vi "chromaSendCommend.vi"(4 "Int_Port Timeout":u32=300, 5 "Clu_RemoteOffsetKeylockResult":T3={"Enum_keyLock"=enum."key board lock Off,recall key lock Off", "Enum_Remote/Local"=enum."Go to Local", "Enum_Offset_Get/Off"=enum."Off", "Clu_Result?"={"Byte"=[FALSE, FALSE, TRUE, FALSE, FALSE, FALSE, FALSE, FALSE], "Step"=1}}, 6 "Clu_SysSetting":T2={"Contrast(1~15)"=7, "Buzzer Volume"=enum."High", "EN50191"=enum."Off", "DC50V AGC"=enum."On", "PassOn(0~100)"=0, "End Of Step"=enum."Off", "EOT"=enum."End Of Test"}, 7 "Clus_STDparameter":T4={"EnumFunnction"=enum."Step Parameters", "Hex_DA"=1, "Hex_Master"=50} {"Hex_DA" format="%x"; "Hex_Master" format="%x"}, 8 "ErrIn":errorcluster, 9 "Clu_PresetParameter":T5, 10 "Clu_StepParameters":T6={"Enum_mode"=enum."AC", "StepIndex(1~10)"=1, "RampTime(100ms)"=20, "DwallTime(100ms)"=0, "TestTime(100ms)"=50, "Falltime(100ms)"=30, "HighLimit(100nA)"=10000, "LowLimit(100nA)"=1000, "ArcLimit(100nA)"=10000, "InrushLimit(100nA)"=0, "Sorce(v)"=1000}) -> (0 "ErrOut":errorcluster, 1 "ChecksumError":bool, 2 "Enum_ErrorType":T1, 3 "Str_ ReplyStr":string)   [LabVIEW 2016]
doc: "Include all commend syntax\nSend a message and receive.check checksum \n\n<b>Clu_RemoteOffsetKeyLockResult: </b>\nKeylock\nRemote/Local\nOffset Get/Off\nResult?\n\n<b>Clus_STDparameter:</b>\nMain parameter of every commend\n\n<b>Clu_syssetting:</b>\ncmd systemsetting\n\n<b>Clu_stepParameters</b>\ncmd stepparameters. use bundle by name to set every parameter\n\n<b>Clu_PresetParameter</b>\ncmd presetparameter\n\n<b>Boolean_comerr\nReturn comport error of not\n\n<b>Boolean_ChecksumCurrect</b>\nmanupulate if check sum is currect or not"
uses:
  TypeDef/Enum_ErrorType.ctl
  meter global.vi
panel:
  out "Time_SendNReceive":u32
  out "Boolean_ComErr":bool
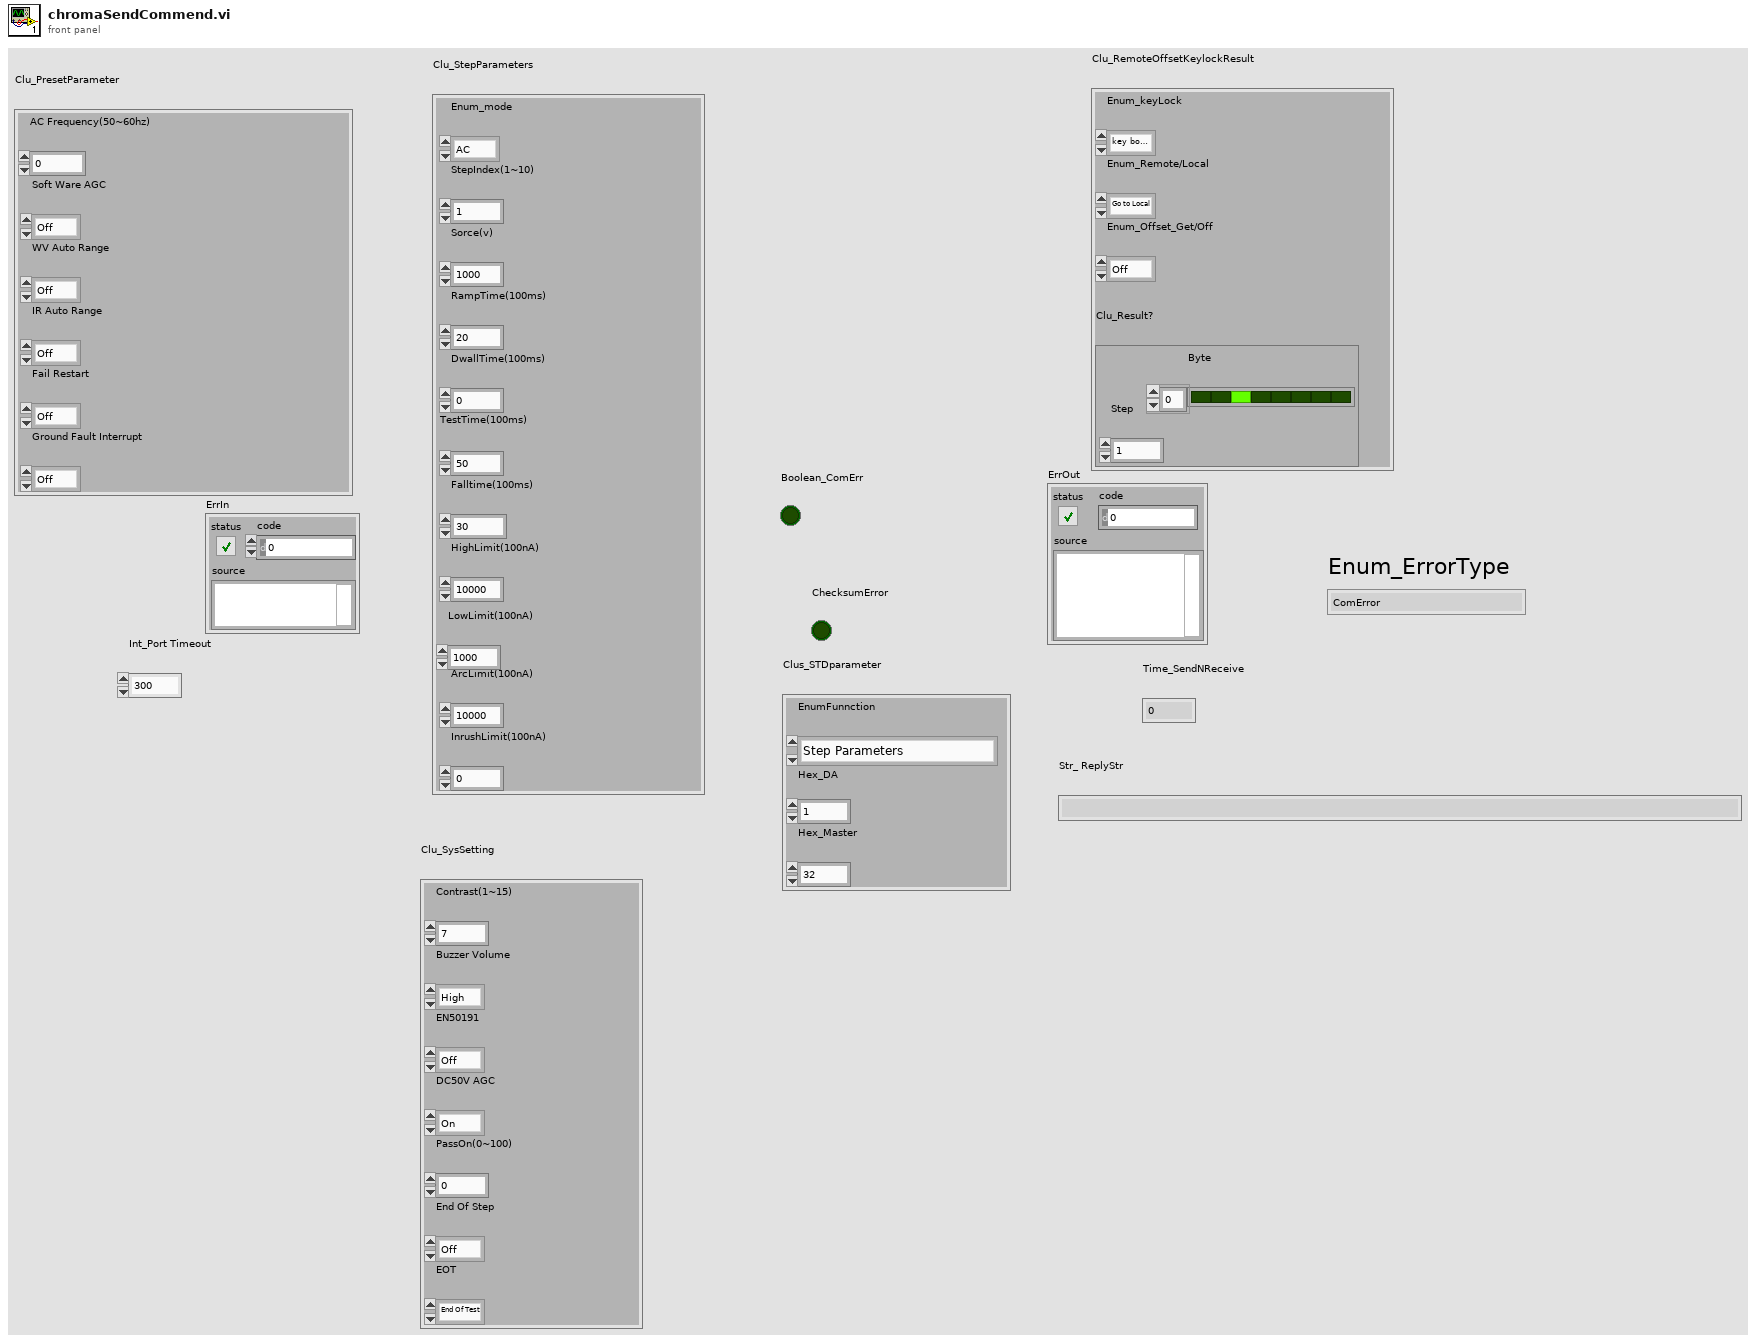
[diagram p1: front panel]
types:
  T1 = typedef "Enum_ErrorType.ctl" = enum16{"ComError", "OK", "Command Error", "Parameter Error"}
  T2 = cluster{"Contrast(1~15)":u8, "Buzzer Volume":enum8{"OFF", "LOW", "Medium", "High"}, "EN50191":enum8{"Off", "On"}, "DC50V AGC":enum8{"Off", "On"}, "PassOn(0~100)":u8, "End Of Step":enum8{"Off", "On"}, "EOT":enum8{"End Of Test", "End Of Timer"}}
  T3 = cluster{"Enum_keyLock":enum8{"key board lock Off,recall key lock Off", "key board lock On,recall key lock Off", "key board lock On,recall key lock On"}, "Enum_Remote/Local":enum8{"Go to Local", "Go to Remote", "Go to Remote and Local Lockout"}, "Enum_Offset_Get/Off":enum8{"Off", "Nonuse", "Get"}, "Clu_Result?":cluster{"Byte":bool[], "Step":u8}}
  T4 = cluster{"EnumFunnction":enum16{"IDN?", "test", "Stop", "Start", "Step Parameters", "Step Patameters?", "Preset Parameter", "Preset parameter?", "Offset Get/Off", "Offset?", "System Setting", "System Setting?", "KeyLock", "KeyLock?", "Initialize All Steps Parameter", "Remote/Local", "Result"}, "Hex_DA":u8, "Hex_Master":u8}
  T5 = cluster{"AC Frequency(50~60hz)":u8, "Soft Ware AGC":enum8{"Off", "On"}, "WV Auto Range":enum8{"Off", "On"}, "IR Auto Range":enum8{"Off", "On"}, "Fail Restart":enum8{"Off", "On"}, "Ground Fault Interrupt":enum8{"Off", "On"}}
  T6 = cluster{"Enum_mode":enum16{"AC", "DC", "IR"}, "StepIndex(1~10)":u8, "RampTime(100ms)":u16, "DwallTime(100ms)":u16, "TestTime(100ms)":u16, "Falltime(100ms)":u16, "HighLimit(100nA)":u32, "LowLimit(100nA)":u32, "ArcLimit(100nA)":u32, "InrushLimit(100nA)":u32, "Sorce(v)":u16}
  T7 = enum8{"Go to Local", "Go to Remote", "Go to Remote and Local Lockout"}
  T8 = enum8{"key board lock Off,recall key lock Off", "key board lock On,recall key lock Off", "key board lock On,recall key lock On"}
  T9 = enum16{"IDN?", "test", "Stop", "Start", "Step Parameters", "Step Patameters?", "Preset Parameter", "Preset parameter?", "Offset Get/Off", "Offset?", "System Setting", "System Setting?", "KeyLock", "KeyLock?", "Initialize All Steps Parameter", "Remote/Local", "Result"}
  T10 = enum16{"big-endian, network order", "native, host order", "little-endian"}
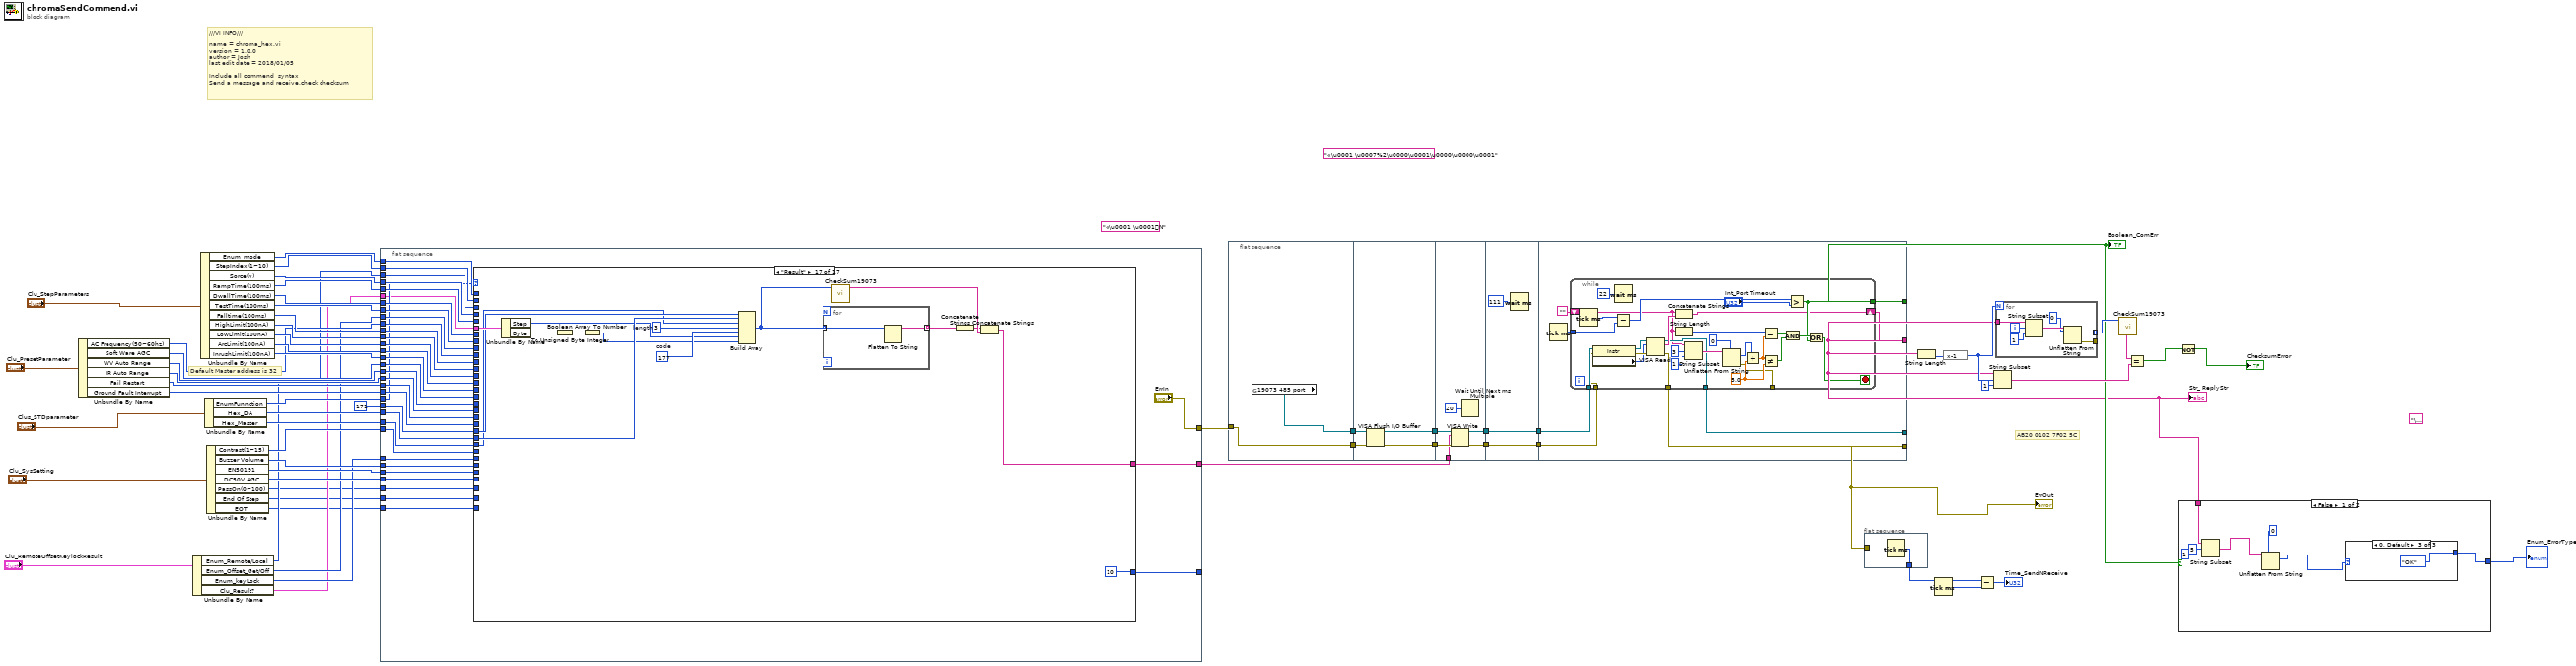
[diagram p0: block diagram]
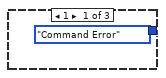
[diagram p2: hidden frame]
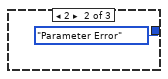
[diagram p3: hidden frame]
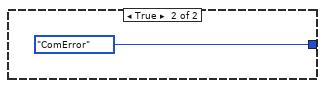
[diagram p4: hidden frame]
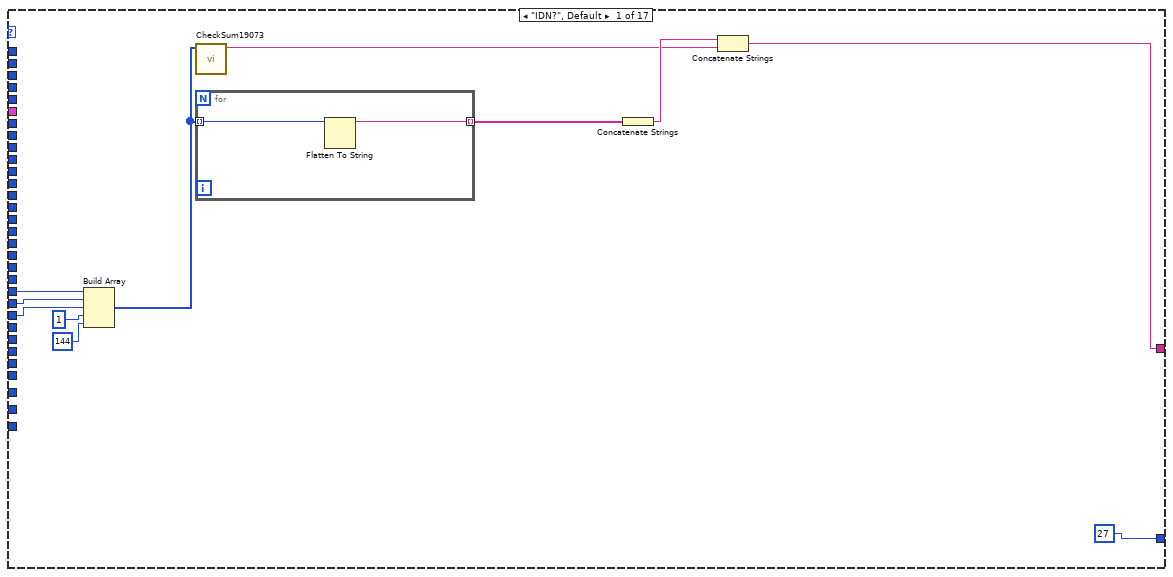
[diagram p5: hidden frame]
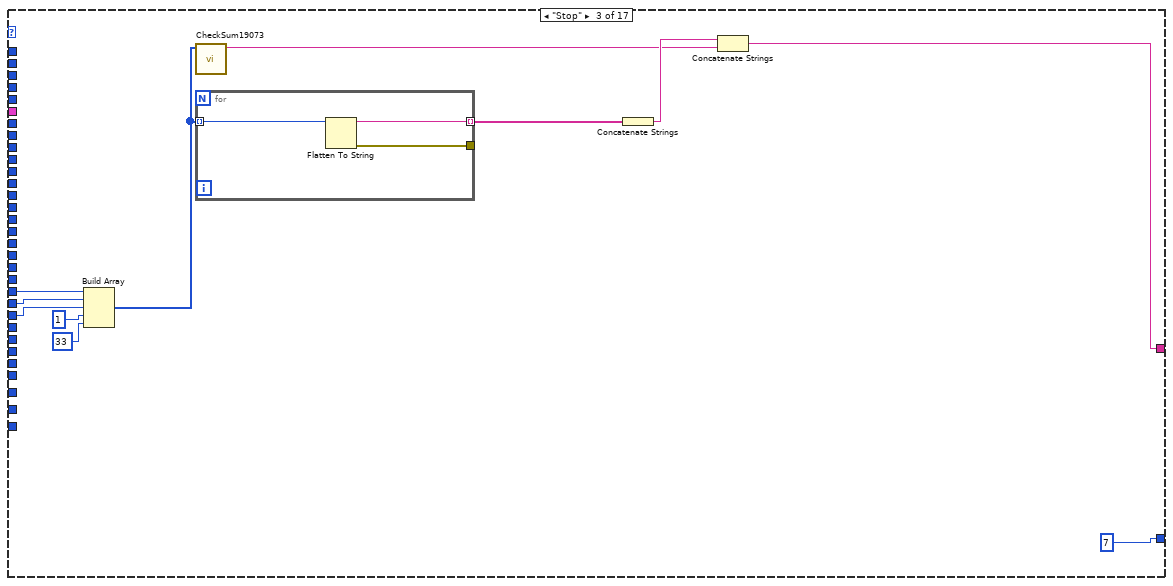
[diagram p7: hidden frame]
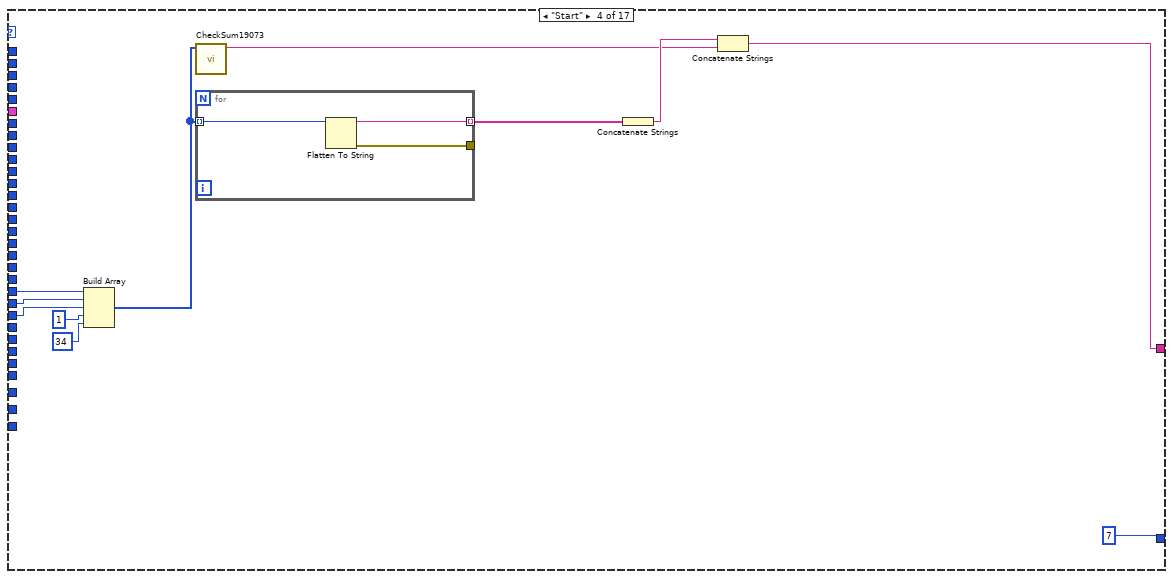
[diagram p8: hidden frame]
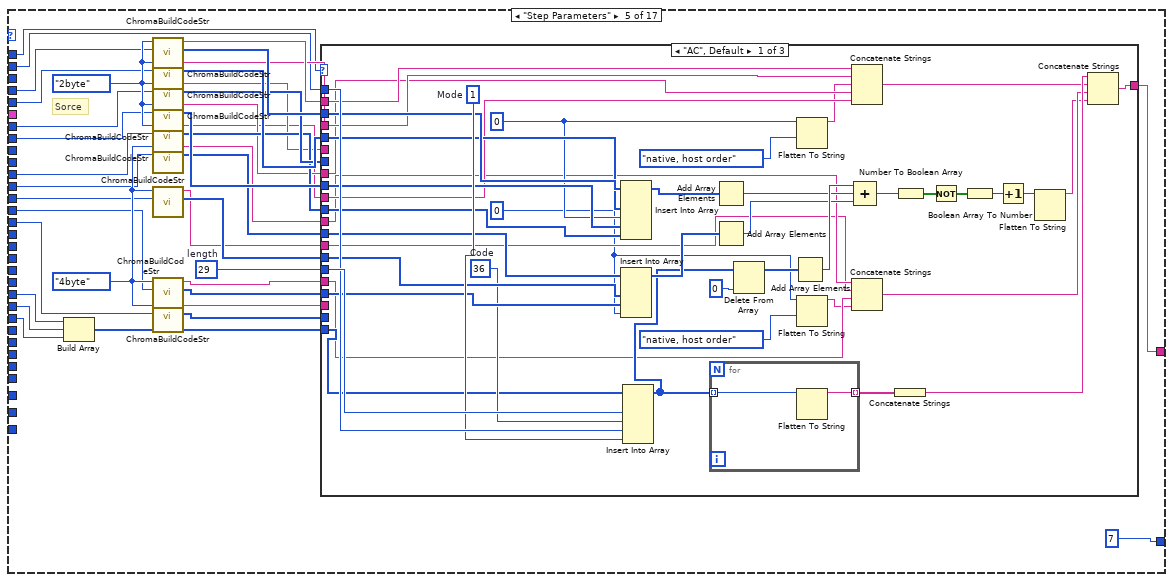
[diagram p9: hidden frame]
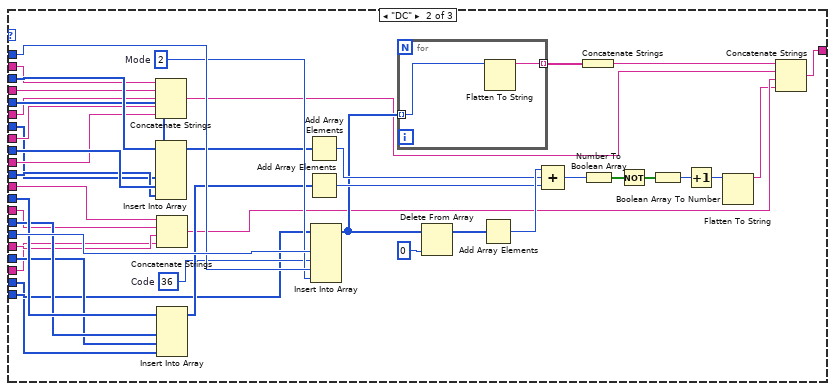
[diagram p10: hidden frame]
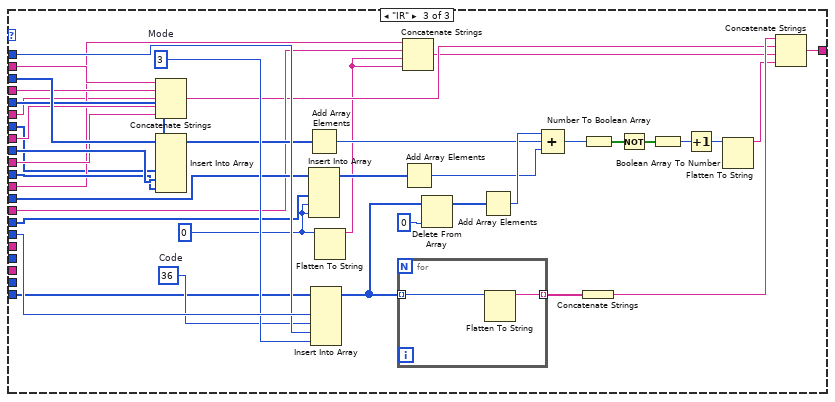
[diagram p11: hidden frame]
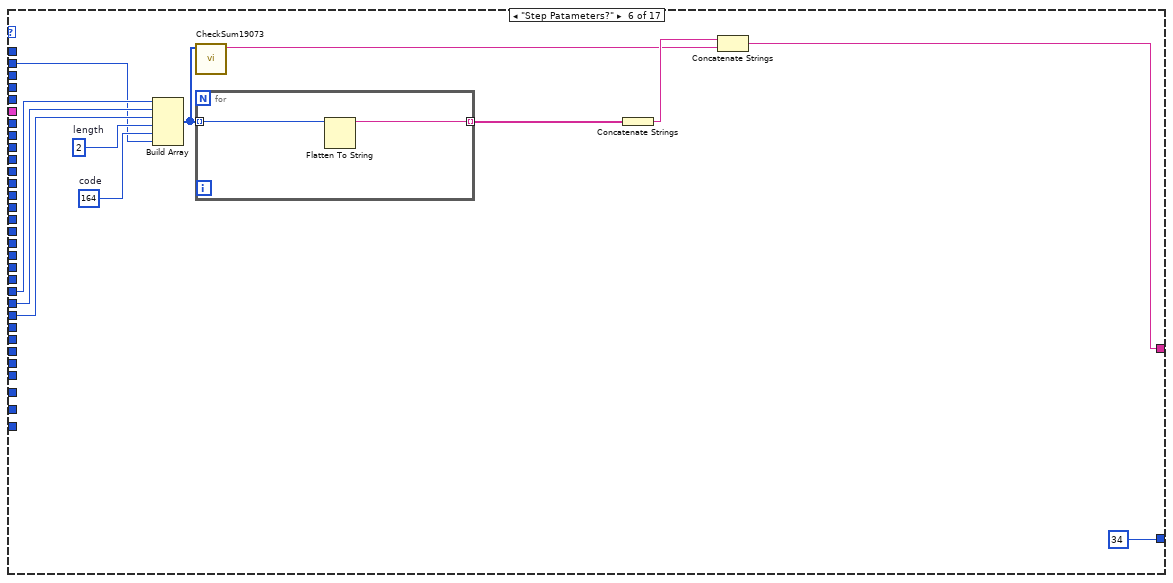
[diagram p12: hidden frame]
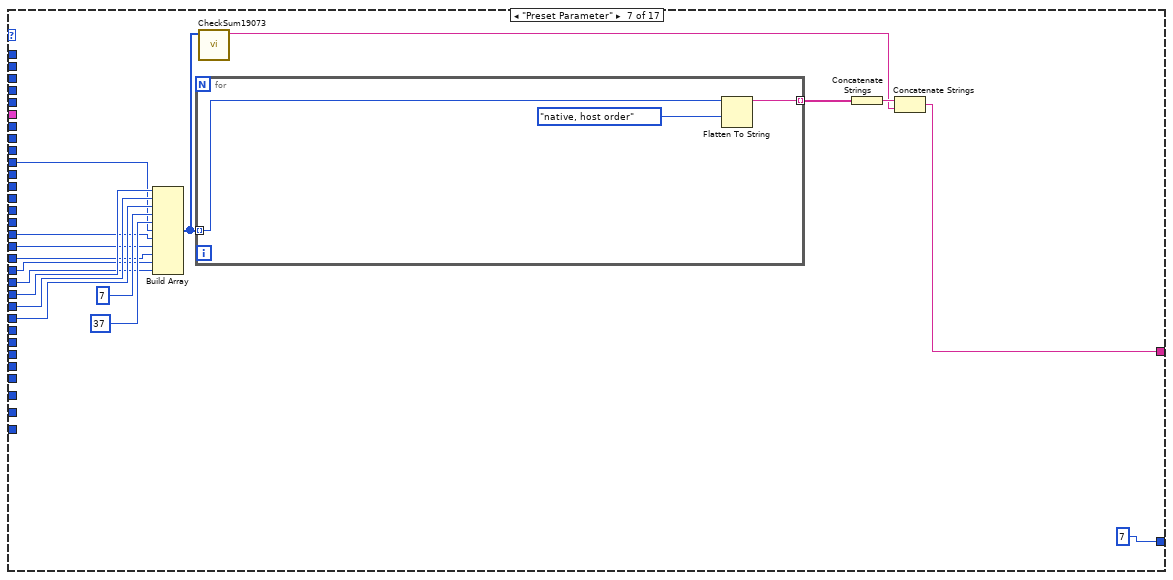
[diagram p13: hidden frame]
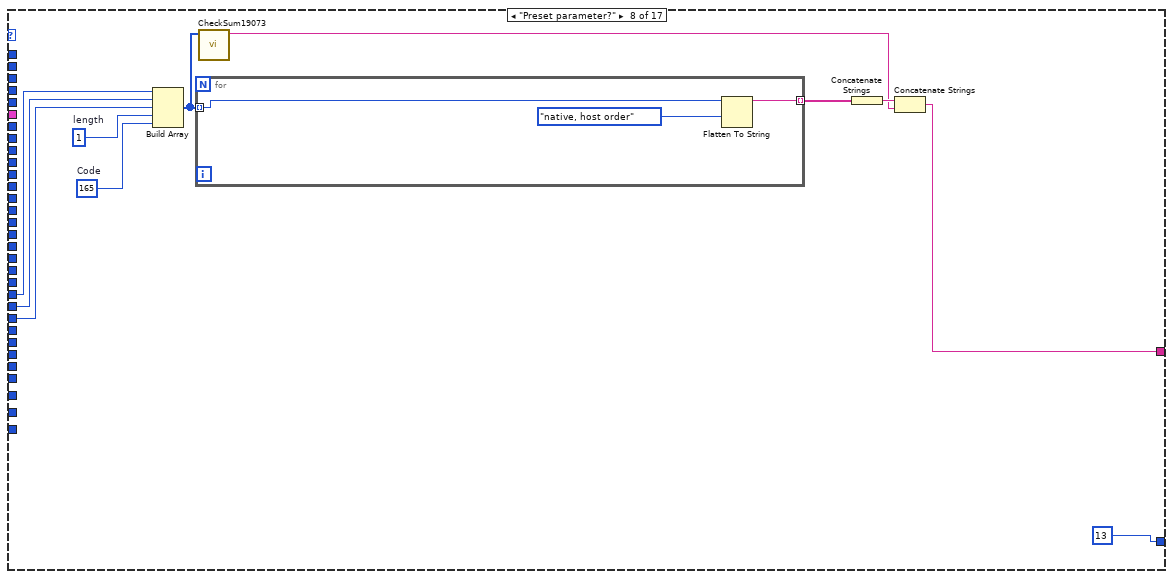
[diagram p14: hidden frame]
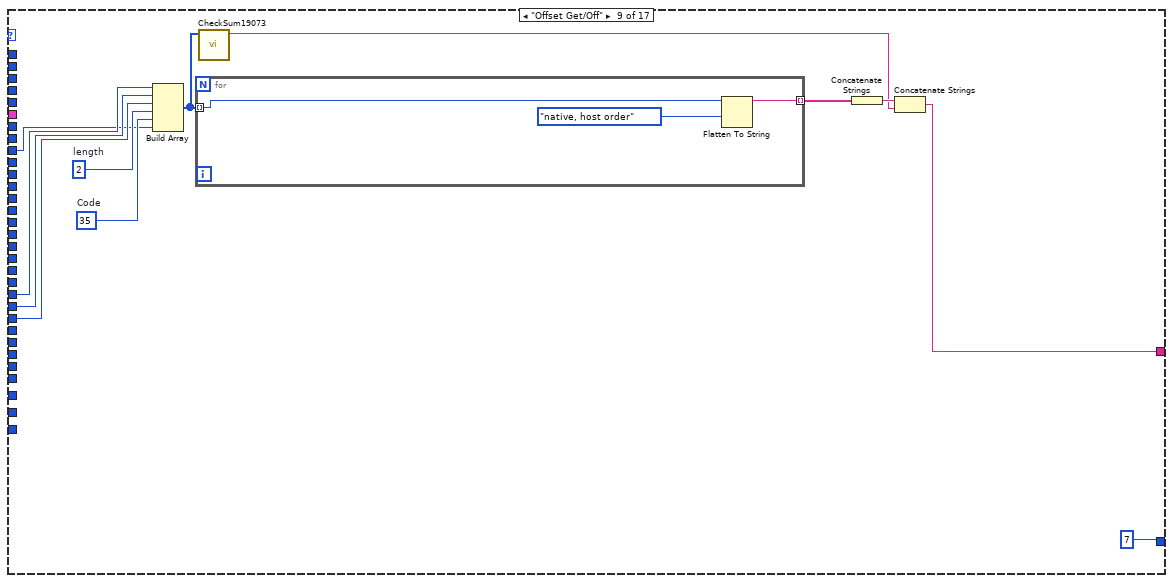
[diagram p15: hidden frame]
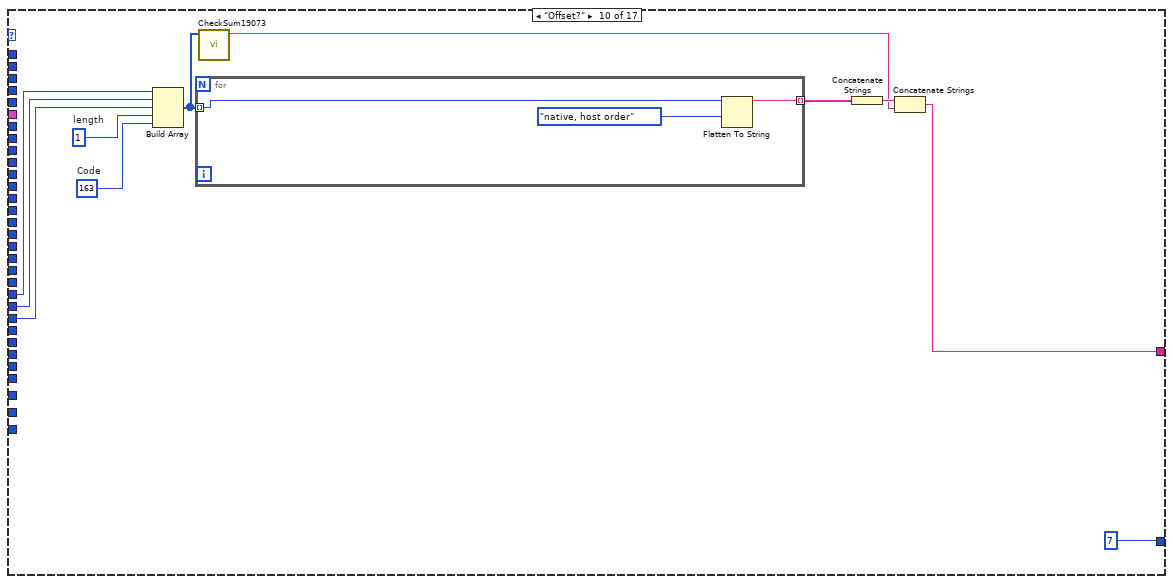
[diagram p16: hidden frame]
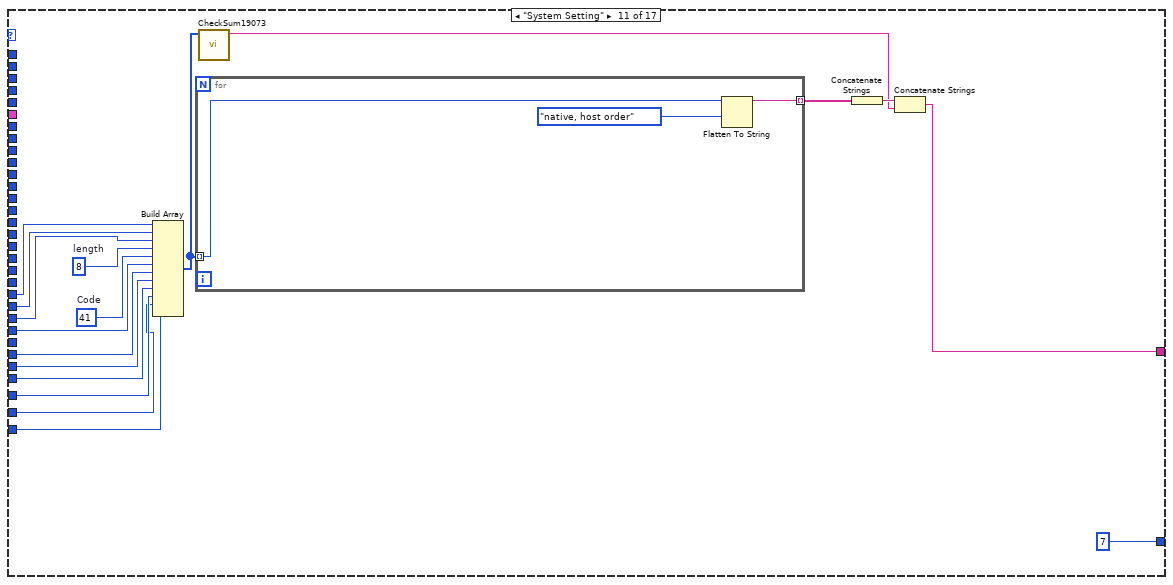
[diagram p17: hidden frame]
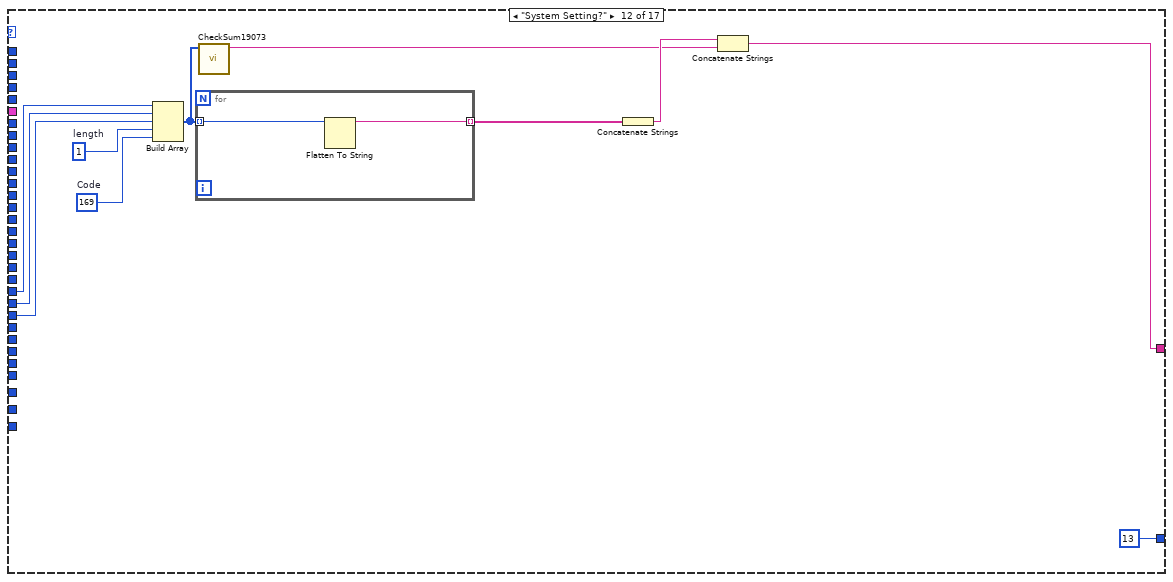
[diagram p18: hidden frame]
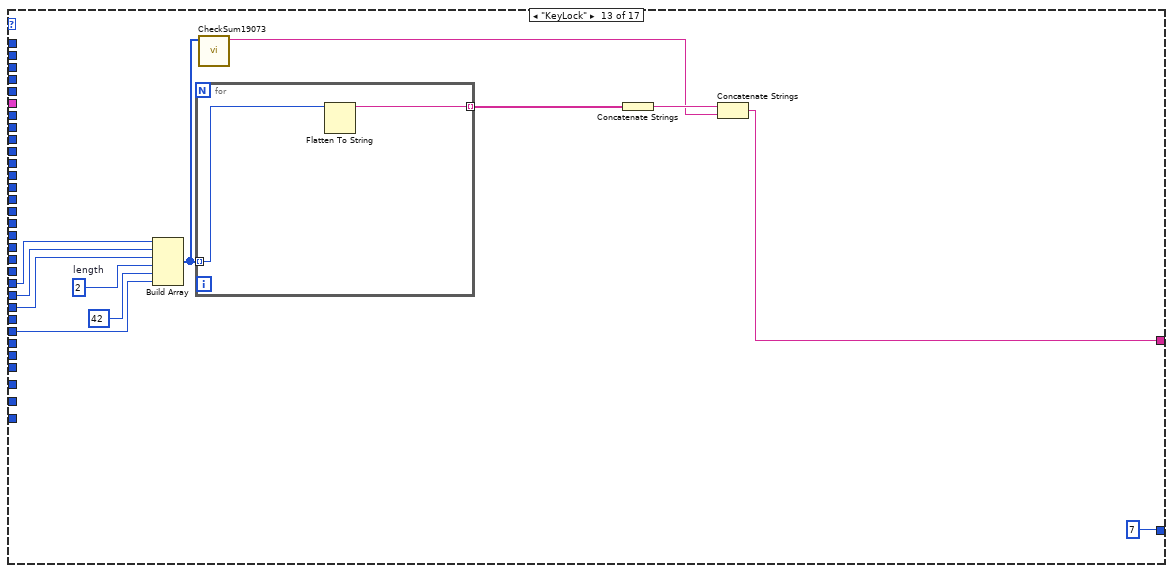
[diagram p19: hidden frame]
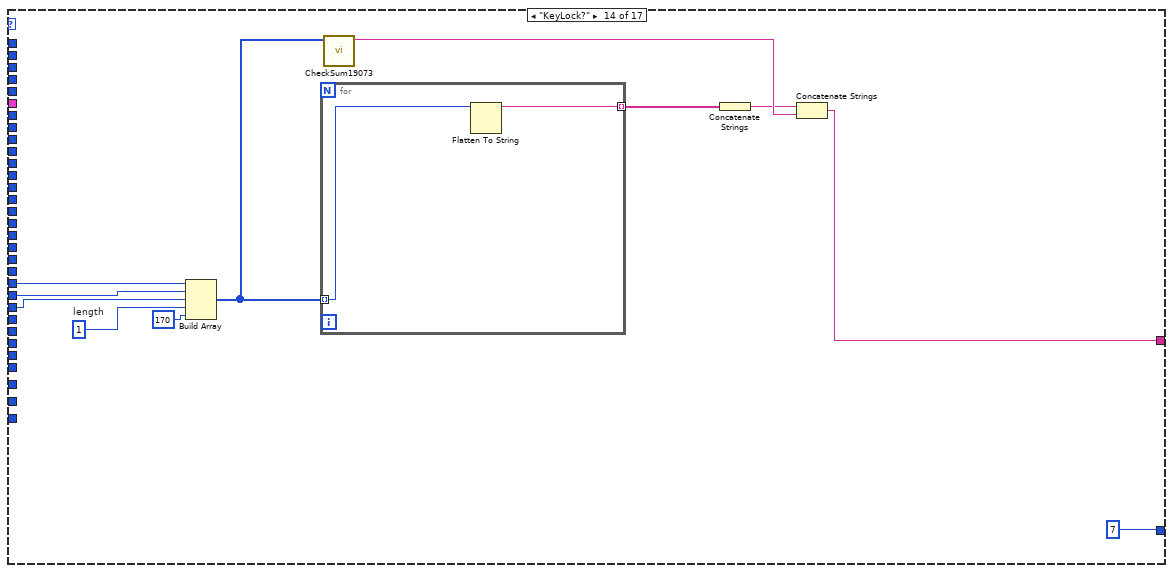
[diagram p20: hidden frame]
diagram:
  (unwired) "\u0002"
  (unwired) "«\u0001 \u0001N" ("Display")
  (unwired) "«\u0001 \u0007%2\u0000\u0001\u0000\u0000\u0001" ("Display")
  # "AB20 0102 7F02 5C"
  # "///VI INFO/// \n\nname = chroma_hex.vi\nversion = 1.0.0\nauthor = Josh\nlast edit date = 2018/01/05\n\nInclude all commend  syntax\nSend a message and receive.check checksum"
  # "Default Master address is 32"
  n1 = Unbundle By Name("Clu_PresetParameter") -> ("AC Frequency(50~60hz)"=w48:u8, "Soft Ware AGC"=w47:enum8{"Off", "On"}, "WV Auto Range"=w46:enum8{"Off", "On"}, "IR Auto Range"=w45:enum8{"Off", "On"}, "Fail Restart"=w44:enum8{"Off", "On"}, "Ground Fault Interrupt"=w43:enum8{"Off", "On"})
  n2 = Unbundle By Name("Clu_RemoteOffsetKeylockResult") -> ("Enum_Remote/Local"=w27:T7, "Enum_Offset_Get/Off"=w26:enum8{"Off", "Nonuse", "Get"}, "Enum_keyLock"=w25:T8, "Clu_Result?"=w21:cluster{"Byte":bool[], "Step":u8})
  n3 = Unbundle By Name("Clu_StepParameters") -> ("Enum_mode"=w60:enum16{"AC", "DC", "IR"}, "StepIndex(1~10)"=w59:u8, "Sorce(v)"=w58:u16, "RampTime(100ms)"=w57:u16, "DwallTime(100ms)"=w56:u16, "TestTime(100ms)"=w55:u16, "Falltime(100ms)"=w54:u16, "HighLimit(100nA)"=w53:u32, "LowLimit(100nA)"=w52:u32, "ArcLimit(100nA)"=w51:u32, "InrushLimit(100nA)"=w50:u32)
  n4 = Unbundle By Name("Clus_STDparameter") -> ("EnumFunnction"=w37:T9, "Hex_DA"=w36:u8, "Hex_Master"=w35:u8)
  n5 = Unbundle By Name("Clu_SysSetting") -> ("Contrast(1~15)"=w42:u8, "Buzzer Volume"=w41:enum8{"OFF", "LOW", "Medium", "High"}, "EN50191"=w40:enum8{"Off", "On"}, "DC50V AGC"=w39:enum8{"Off", "On"}, "PassOn(0~100)"=w19:u8, "End Of Step"=w18:enum8{"Off", "On"}, "EOT"=w17:enum8{"End Of Test", "End Of Timer"})
  n6 = flat-sequence {
    tunnel: u8 171 -> [w97]
    tunnel: w60 -> [w96]
    tunnel: w59 -> [w95]
    tunnel: w58 -> [w94]
    tunnel: w57 -> [w93]
    tunnel: w56 -> [w92]
    tunnel: w55 -> [w91]
    tunnel: w54 -> [w90]
    tunnel: w53 -> [w89]
    tunnel: w52 -> [w88]
    tunnel: w51 -> [w87]
    tunnel: w50 -> [w86]
    tunnel: w48 -> [w85]
    tunnel: w47 -> [w84]
    tunnel: w46 -> [w83]
    tunnel: w45 -> [w82]
    tunnel: w44 -> [w81]
    tunnel: w43 -> [w80]
    tunnel: w26 -> [w79]
    tunnel: w42 -> [w78]
    tunnel: w41 -> [w77]
    tunnel: w40 -> [w76]
    tunnel: w39 -> [w75]
    tunnel: w25 -> [w74]
    tunnel: w27 -> [w73]
    tunnel: w37 -> [w72]
    tunnel: w36 -> [w71]
    tunnel: w35 -> [w70]
    tunnel: w21 -> [w69]
    tunnel: [w68] -> w30
    tunnel: ["ErrIn"] -> w29
    tunnel: [w66] -> _
    tunnel: w19 -> [w65]
    tunnel: w18 -> [w64]
    tunnel: w17 -> [w63]
    frame #0 {
      n7 = case shown="\"Result\"" w72 {
        tunnel: w71 -> [w108 _ w120 w128 w175 w319 w338 w352 w367 w381 w402 w416 w430 w441 w454 w468 w486]
        tunnel: w70 -> [w107 _ w119 w127 w174 w318 w337 w351 w366 w380 w401 w415 w429 w440 w453 w467 w485]
        tunnel: [w102 _ w112 w126 w151 w310 w324 w344 w358 w373 w390 w408 w421 w435 w448 w461 w475] -> w68
        tunnel: w97 -> [w100 _ w121 w129 w176 w320 w339 w353 w368 w382 w403 w417 w431 w442 w455 w469 w487]
        tunnel: w96 -> [_ _ _ _ w150 _ _ _ _ _ _ _ _ _ _ _ _]
        tunnel: w95 -> [_ _ _ _ w149 w315 _ _ _ _ _ _ _ _ _ _ _]
        tunnel: w94 -> [_ _ _ _ w148 _ _ _ _ _ _ _ _ _ _ _ _]
        tunnel: w93 -> [_ _ _ _ w147 _ _ _ _ _ _ _ _ _ _ _ _]
        tunnel: w92 -> [_ _ _ _ w146 _ _ _ _ _ _ _ _ _ _ _ _]
        tunnel: w91 -> [_ _ _ _ w145 _ _ _ _ _ _ _ _ _ _ _ _]
        tunnel: w90 -> [_ _ _ _ w144 _ _ _ _ _ _ _ _ _ _ _ _]
        tunnel: w89 -> [_ _ _ _ w143 _ _ _ _ _ _ _ _ _ _ _ _]
        tunnel: w88 -> [_ _ _ _ w142 _ _ _ _ _ _ _ _ _ _ _ _]
        tunnel: w87 -> [_ _ _ _ w141 _ _ _ _ _ _ _ _ _ _ _ _]
        tunnel: w86 -> [_ _ _ _ w140 _ _ _ _ _ _ _ _ _ _ _ _]
        tunnel: w85 -> [_ _ _ _ _ _ w334 _ _ _ _ _ _ _ _ _ _]
        tunnel: w84 -> [_ _ _ _ _ _ w333 _ _ _ _ _ _ _ _ _ _]
        tunnel: w83 -> [_ _ _ _ _ _ w332 _ _ _ _ _ _ _ _ _ _]
        tunnel: w82 -> [_ _ _ _ _ _ w331 _ _ _ _ _ _ _ _ _ _]
        tunnel: w81 -> [_ _ _ _ _ _ w330 _ _ _ _ _ _ _ _ _ _]
        tunnel: w80 -> [_ _ _ _ _ _ w329 _ _ _ _ _ _ _ _ _ _]
        tunnel: w79 -> [_ _ _ _ _ _ _ _ w363 _ _ _ _ _ _ _ _]
        tunnel: w78 -> [_ _ _ _ _ _ _ _ _ _ w398 _ _ _ _ _ _]
        tunnel: w77 -> [_ _ _ _ _ _ _ _ _ _ w397 _ _ _ _ _ _]
        tunnel: w76 -> [_ _ _ _ _ _ _ _ _ _ w396 _ _ _ _ _ _]
        tunnel: w75 -> [_ _ _ _ _ _ _ _ _ _ w395 _ _ _ _ _ _]
        tunnel: w74 -> [_ _ _ _ _ _ _ _ _ _ _ _ w426 _ _ _ _]
        tunnel: w73 -> [_ _ _ _ _ _ _ _ _ _ _ _ _ _ _ w466 _]
        tunnel: w69 -> [_ _ _ _ _ _ _ _ _ _ _ _ _ _ _ _ w489]
        tunnel: [27 _ 7 7 7 34 7 13 7 7 7 13 7 7 7 7 10] -> w66
        tunnel: w65 -> [_ _ _ _ _ _ _ _ _ _ w388 _ _ _ _ _ _]
        tunnel: w64 -> [_ _ _ _ _ _ _ _ _ _ w387 _ _ _ _ _ _]
        tunnel: w63 -> [_ _ _ _ _ _ _ _ _ _ w386 _ _ _ _ _ _]
        frame "IDN?", Default {
          n8 = Build Array(w100, w108, w107, u8 1, u8 144) -> (w99:u8[])
          n9 = call "CheckSum19073.vi"("Array"=w99) -> ("data string"=w103:string)  [unwired: 10 in]
          n10 = for {
            tunnel: [w110] -> w105 mode=indexing
            tunnel: w99 -> [w109] mode=indexing
            n11 = Flatten To String(anything=w109) -> (data string=w110:string)  [unwired: 3 in, 2 out]
          }
          n12 = Concatenate Strings(w105) -> (w104:string)
          n13 = Concatenate Strings(w104, w103) -> (w102:string)
        }
        frame "test" {
        }
        frame "Stop" {
          n14 = Build Array(w121, w120, w119, u8 1, u8 33) -> (w116:u8[])
          n15 = call "CheckSum19073.vi"("Array"=w116) -> ("data string"=w113:string)  [unwired: 10 in]
          n16 = for {
            tunnel: w116 -> [w124] mode=indexing
            tunnel: [w123] -> _
            tunnel: [w122] -> w115 mode=indexing
            n17 = Flatten To String(anything=w124) -> (data string=w122:string, error out=w123:errorcluster)  [unwired: 3 in, 1 out]
          }
          n18 = Concatenate Strings(w115) -> (w114:string)
          n19 = Concatenate Strings(w114, w113) -> (w112:string)
        }
        frame "Start" {
          n20 = Build Array(w129, w128, w127, u8 1, u8 34) -> (w133:u8[])
          n21 = call "CheckSum19073.vi"("Array"=w133) -> ("data string"=w130:string)  [unwired: 10 in]
          n22 = for {
            tunnel: w133 -> [w138] mode=indexing
            tunnel: [w137] -> _
            tunnel: [w136] -> w132 mode=indexing
            n23 = Flatten To String(anything=w138) -> (data string=w136:string, error out=w137:errorcluster)  [unwired: 3 in, 1 out]
          }
          n24 = Concatenate Strings(w132) -> (w131:string)
          n25 = Concatenate Strings(w131, w130) -> (w126:string)
        }
        frame "Step Parameters" {
          w162 = enum16{"1byte", "2byte", "4byte"}."4byte" ("Enum_datatype")
          w167 = enum16{"1byte", "2byte", "4byte"}."2byte" ("Enum_datatype")
          w172 = u8 29  # length
          # "Sorce"
          n26 = Build Array(w176, w175, w174) -> (w173:u8[])
          n27 = call "ChromaBuildCodeStr.vi"("Hex_input"=w148, "Enum_datatype"=w167) -> ("Array"=w171:u8[], "data string"=w160:string)  [unwired: 8 in]
          n28 = call "ChromaBuildCodeStr.vi"("Hex_input"=w147, "Enum_datatype"=w167) -> ("Array"=w170:u8[], "data string"=w159:string)  [unwired: 8 in]
          n29 = call "ChromaBuildCodeStr.vi"("Hex_input"=w146, "Enum_datatype"=w167) -> ("Array"=w169:u8[], "data string"=w158:string)  [unwired: 8 in]
          n30 = call "ChromaBuildCodeStr.vi"("Hex_input"=w145, "Enum_datatype"=w167) -> ("Array"=w168:u8[], "data string"=w157:string)  [unwired: 8 in]
          n31 = call "ChromaBuildCodeStr.vi"("Hex_input"=w144, "Enum_datatype"=w167) -> ("Array"=w166:u8[], "data string"=w156:string)  [unwired: 8 in]
          n32 = call "ChromaBuildCodeStr.vi"("Hex_input"=w143, "Enum_datatype"=w162) -> ("Array"=w165:u8[], "data string"=w155:string)  [unwired: 8 in]
          n33 = call "ChromaBuildCodeStr.vi"("Hex_input"=w142, "Enum_datatype"=w162) -> ("Array"=w164:u8[], "data string"=w154:string)  [unwired: 8 in]
          n34 = call "ChromaBuildCodeStr.vi"("Hex_input"=w141, "Enum_datatype"=w162) -> ("Array"=w163:u8[], "data string"=w153:string)  [unwired: 8 in]
          n35 = call "ChromaBuildCodeStr.vi"("Hex_input"=w140, "Enum_datatype"=w162) -> ("Array"=w161:u8[], "data string"=w152:string)  [unwired: 8 in]
          n36 = case shown="\"AC\", Default" w150 {
            tunnel: w173 -> [w198 w242 w285]
            tunnel: w172 -> [w217 w261 w303]
            tunnel: w171 -> [w214 w258 w300]
            tunnel: w170 -> [w213 w257 w299]
            tunnel: w149 -> [w216 w260 w302]
            tunnel: w169 -> [_ w223 w269]
            tunnel: w168 -> [w212 w256 w298]
            tunnel: w166 -> [w211 w255 w297]
            tunnel: w165 -> [w209 w253 w295]
            tunnel: w164 -> [w208 w252 w294]
            tunnel: w163 -> [w207 w251 _]
            tunnel: w161 -> [_ w226 _]
            tunnel: w160 -> [w194 w238 w281]
            tunnel: w159 -> [w193 w237 w280]
            tunnel: w158 -> [_ w224 w270]
            tunnel: w157 -> [w192 w236 w279]
            tunnel: w156 -> [w191 w235 w278]
            tunnel: w155 -> [w187 w234 w277]
            tunnel: w154 -> [w186 w233 w276]
            tunnel: w153 -> [w185 w232 _]
            tunnel: w152 -> [_ w225 _]
            tunnel: [w177 w227 w271] -> w151
            frame "AC", Default {
              w184 = u32 0
              w190 = u16 0
              w215 = u8 1  # Mode
              w201 = u8 36  # Code
              n37 = Insert Into Array(array=w214, new element #1=w213, new element #2=w190, new element #3=w212, new element #4=w211) -> (w210:u8[])  [unwired: 1 in]
              n38 = Insert Into Array(array=w209, new element #1=w208, new element #2=w207, new element #3=w184) -> (w206:u8[])  [unwired: 1 in]
              n39 = Insert Into Array(array=w198, new element #1=w217, new element #2=w201, new element #3=w216, new element #4=w215) -> (w197:u8[])  [unwired: 1 in]
              n40 = for {
                tunnel: w197 -> [w222] mode=indexing
                tunnel: [w221] -> w199 mode=indexing
                n41 = Flatten To String(anything=w222) -> (data string=w221:string)  [unwired: 3 in, 2 out]
              }
              n42 = Add Array Elements(numeric array=w210) -> (sum=w204:u8)
              n43 = Add Array Elements(numeric array=w206) -> (sum=w203:u8)
              n44 = Delete From Array(array=w197, index=0) -> (array with subset deleted=w195:u8[])  [unwired: 1 in, 1 out]
              n45 = Add Array Elements(numeric array=w195) -> (sum=w205:u8)
              n46 = Flatten To String(anything=w190, byte order (0:big-endian, network order)=T10."native, host order") -> (data string=w188:string)  [unwired: 2 in, 2 out]
              n47 = Flatten To String(anything=w184, byte order (0:big-endian, network order)=T10."native, host order") -> (data string=w182:string)  [unwired: 2 in, 2 out]
              n48 = Concatenate Strings(w194, w193, w188, w192, w191) -> (w180:string)
              n49 = Concatenate Strings(w187, w186, w185, w182) -> (w179:string)
              n50 = Compound Arithmetic op=ADD(w205, w204, w203) -> (w202:u8)
              n51 = Concatenate Strings(w199) -> (w181:string)
              n52 = Number To Boolean Array(number=w202) -> (Boolean array=w220:bool[])
              n53 = Not(x=w220) -> (.not. x?=w219:bool[])
              n54 = Boolean Array To Number(Boolean array=w219) -> (number=w218:u32)
              n55 = Increment(x=w218) -> (x+1=w200:u8)
              n56 = Flatten To String(anything=w200) -> (data string=w178:string)  [unwired: 3 in, 2 out]
              n57 = Concatenate Strings(w181, w180, w179, w178) -> (w177:string)
            }
            frame "DC" {
              w259 = u8 2  # Mode
              w245 = u8 36  # Code
              n58 = Concatenate Strings(w238, w237, w224, w236, w235) -> (w230:string)
              n59 = Insert Into Array(array=w258, new element #1=w257, new element #2=w223, new element #3=w256, new element #4=w255) -> (w254:u8[])  [unwired: 1 in]
              n60 = Concatenate Strings(w234, w233, w232, w225) -> (w229:string)
              n61 = Insert Into Array(array=w253, new element #1=w252, new element #2=w251, new element #3=w226) -> (w250:u8[])  [unwired: 1 in]
              n62 = Add Array Elements(numeric array=w254) -> (sum=w248:u8)
              n63 = Add Array Elements(numeric array=w250) -> (sum=w247:u8)
              n64 = Insert Into Array(array=w242, new element #1=w261, new element #2=w245, new element #3=w260, new element #4=w259) -> (w241:u8[])  [unwired: 1 in]
              n65 = for {
                tunnel: w241 -> [w266] mode=indexing
                tunnel: [w265] -> w243 mode=indexing
                n66 = Flatten To String(anything=w266) -> (data string=w265:string)  [unwired: 3 in, 2 out]
              }
              n67 = Delete From Array(array=w241, index=0) -> (array with subset deleted=w239:u8[])  [unwired: 1 in, 1 out]
              n68 = Add Array Elements(numeric array=w239) -> (sum=w249:u8)
              n69 = Compound Arithmetic op=ADD(w249, w248, w247) -> (w246:u8)
              n70 = Concatenate Strings(w243) -> (w231:string)
              n71 = Number To Boolean Array(number=w246) -> (Boolean array=w264:bool[])
              n72 = Not(x=w264) -> (.not. x?=w263:bool[])
              n73 = Boolean Array To Number(Boolean array=w263) -> (number=w262:u32)
              n74 = Increment(x=w262) -> (x+1=w244:u8)
              n75 = Flatten To String(anything=w244) -> (data string=w228:string)  [unwired: 3 in, 2 out]
              n76 = Concatenate Strings(w231, w230, w229, w228) -> (w227:string)
            }
            frame "IR" {
              w268 = u32 0
              w301 = 3  # Mode
              w288 = u8 36  # Code
              n77 = Concatenate Strings(w281, w280, w270, w279, w278) -> (w274:string)
              n78 = Insert Into Array(array=w300, new element #1=w299, new element #2=w269, new element #3=w298, new element #4=w297) -> (w296:u8[])  [unwired: 1 in]
              n79 = Add Array Elements(numeric array=w296) -> (sum=w291:u8)
              n80 = Insert Into Array(array=w295, new element #1=w294, new element #2=w268, new element #3=w268) -> (w293:u8[])  [unwired: 1 in]
              n81 = Insert Into Array(array=w285, new element #1=w303, new element #2=w288, new element #3=w302, new element #4=w301) -> (w284:u8[])  [unwired: 1 in]
              n82 = Flatten To String(anything=w268) -> (data string=w267:string)  [unwired: 3 in, 2 out]
              n83 = for {
                tunnel: w284 -> [w308] mode=indexing
                tunnel: [w307] -> w286 mode=indexing
                n84 = Flatten To String(anything=w308) -> (data string=w307:string)  [unwired: 3 in, 2 out]
              }
              n85 = Concatenate Strings(w277, w276, w267, w267) -> (w273:string)
              n86 = Add Array Elements(numeric array=w293) -> (sum=w290:u8)
              n87 = Delete From Array(array=w284, index=0) -> (array with subset deleted=w282:u8[])  [unwired: 1 in, 1 out]
              n88 = Add Array Elements(numeric array=w282) -> (sum=w292:u8)
              n89 = Compound Arithmetic op=ADD(w292, w291, w290) -> (w289:u8)
              n90 = Concatenate Strings(w286) -> (w275:string)
              n91 = Number To Boolean Array(number=w289) -> (Boolean array=w306:bool[])
              n92 = Not(x=w306) -> (.not. x?=w305:bool[])
              n93 = Boolean Array To Number(Boolean array=w305) -> (number=w304:u32)
              n94 = Increment(x=w304) -> (x+1=w287:u8)
              n95 = Flatten To String(anything=w287) -> (data string=w272:string)  [unwired: 3 in, 2 out]
              n96 = Concatenate Strings(w275, w274, w273, w272) -> (w271:string)
            }
          }
        }
        frame "Step Patameters?" {
          w316 = u8 164  # code
          w317 = u8 2  # length
          n97 = Build Array(w320, w319, w318, w317, w316, w315) -> (w314:u8[])
          n98 = call "CheckSum19073.vi"("Array"=w314) -> ("data string"=w311:string)  [unwired: 10 in]
          n99 = for {
            tunnel: w314 -> [w322] mode=indexing
            tunnel: [w321] -> w313 mode=indexing
            n100 = Flatten To String(anything=w322) -> (data string=w321:string)  [unwired: 3 in, 2 out]
          }
          n101 = Concatenate Strings(w313) -> (w312:string)
          n102 = Concatenate Strings(w312, w311) -> (w310:string)
        }
        frame "Preset Parameter" {
          n103 = Build Array(w339, w338, w337, u8 7 ("length"), u8 37, w334, w333, w332, w331, w330, w329) -> (w328:u8[])
          n104 = for {
            tunnel: w328 -> [w342] mode=indexing
            tunnel: [w340] -> w327 mode=indexing
            n105 = Flatten To String(anything=w342, byte order (0:big-endian, network order)=T10."native, host order") -> (data string=w340:string)  [unwired: 2 in, 2 out]
          }
          n106 = call "CheckSum19073.vi"("Array"=w328) -> ("data string"=w325:string)  [unwired: 10 in]
          n107 = Concatenate Strings(w327) -> (w326:string)
          n108 = Concatenate Strings(w326, w325) -> (w324:string)
        }
        frame "Preset parameter?" {
          w349 = u8 165  # Code
          w350 = u8 1  # length
          n109 = Build Array(w353, w352, w351, w350, w349) -> (w348:u8[])
          n110 = for {
            tunnel: w348 -> [w356] mode=indexing
            tunnel: [w354] -> w347 mode=indexing
            n111 = Flatten To String(anything=w356, byte order (0:big-endian, network order)=T10."native, host order") -> (data string=w354:string)  [unwired: 2 in, 2 out]
          }
          n112 = call "CheckSum19073.vi"("Array"=w348) -> ("data string"=w345:string)  [unwired: 10 in]
          n113 = Concatenate Strings(w347) -> (w346:string)
          n114 = Concatenate Strings(w346, w345) -> (w344:string)
        }
        frame "Offset Get/Off" {
          w364 = u8 35  # Code
          w365 = u8 2  # length
          n115 = Build Array(w368, w367, w366, w365, w364, w363) -> (w362:u8[])
          n116 = for {
            tunnel: w362 -> [w371] mode=indexing
            tunnel: [w369] -> w361 mode=indexing
            n117 = Flatten To String(anything=w371, byte order (0:big-endian, network order)=T10."native, host order") -> (data string=w369:string)  [unwired: 2 in, 2 out]
          }
          n118 = call "CheckSum19073.vi"("Array"=w362) -> ("data string"=w359:string)  [unwired: 10 in]
          n119 = Concatenate Strings(w361) -> (w360:string)
          n120 = Concatenate Strings(w360, w359) -> (w358:string)
        }
        frame "Offset?" {
          w378 = u8 163  # Code
          w379 = u8 1  # length
          n121 = Build Array(w382, w381, w380, w379, w378) -> (w377:u8[])
          n122 = for {
            tunnel: w377 -> [w385] mode=indexing
            tunnel: [w383] -> w376 mode=indexing
            n123 = Flatten To String(anything=w385, byte order (0:big-endian, network order)=T10."native, host order") -> (data string=w383:string)  [unwired: 2 in, 2 out]
          }
          n124 = call "CheckSum19073.vi"("Array"=w377) -> ("data string"=w374:string)  [unwired: 10 in]
          n125 = Concatenate Strings(w376) -> (w375:string)
          n126 = Concatenate Strings(w375, w374) -> (w373:string)
        }
        frame "System Setting" {
          w399 = u8 41  # Code
          w400 = u8 8  # length
          n127 = Build Array(w403, w402, w401, w400, w399, w398, w397, w396, w395, w388, w387, w386) -> (w394:u8[])
          n128 = for {
            tunnel: w394 -> [w406] mode=indexing
            tunnel: [w404] -> w392 mode=indexing
            n129 = Flatten To String(anything=w406, byte order (0:big-endian, network order)=T10."native, host order") -> (data string=w404:string)  [unwired: 2 in, 2 out]
          }
          n130 = call "CheckSum19073.vi"("Array"=w394) -> ("data string"=w391:string)  [unwired: 10 in]
          n131 = Concatenate Strings(w392) -> (w393:string)
          n132 = Concatenate Strings(w393, w391) -> (w390:string)
        }
        frame "System Setting?" {
          w413 = u8 169  # Code
          w414 = u8 1  # length
          n133 = Build Array(w417, w416, w415, w414, w413) -> (w412:u8[])
          n134 = for {
            tunnel: w412 -> [w419] mode=indexing
            tunnel: [w418] -> w411 mode=indexing
            n135 = Flatten To String(anything=w419) -> (data string=w418:string)  [unwired: 3 in, 2 out]
          }
          n136 = call "CheckSum19073.vi"("Array"=w412) -> ("data string"=w409:string)  [unwired: 10 in]
          n137 = Concatenate Strings(w411) -> (w410:string)
          n138 = Concatenate Strings(w410, w409) -> (w408:string)
        }
        frame "KeyLock" {
          w428 = u8 2  # length
          n139 = Build Array(w431, w430, w429, w428, u8 42, w426) -> (w422:u8[])
          n140 = for {
            tunnel: w422 -> [w433] mode=indexing
            tunnel: [w432] -> w425 mode=indexing
            n141 = Flatten To String(anything=w433) -> (data string=w432:string)  [unwired: 3 in, 2 out]
          }
          n142 = call "CheckSum19073.vi"("Array"=w422) -> ("data string"=w423:string)  [unwired: 10 in]
          n143 = Concatenate Strings(w425) -> (w424:string)
          n144 = Concatenate Strings(w424, w423) -> (w421:string)
        }
        frame "KeyLock?" {
          w444 = u8 1  # length
          n145 = Build Array(w442, w441, w440, w444, u8 170 ("code")) -> (w436:u8[])
          n146 = for {
            tunnel: w436 -> [w446] mode=indexing
            tunnel: [w445] -> w437 mode=indexing
            n147 = Flatten To String(anything=w446) -> (data string=w445:string)  [unwired: 3 in, 2 out]
          }
          n148 = call "CheckSum19073.vi"("Array"=w436) -> ("data string"=w439:string)  [unwired: 10 in]
          n149 = Concatenate Strings(w437) -> (w438:string)
          n150 = Concatenate Strings(w438, w439) -> (w435:string)
        }
        frame "Initialize All Steps Parameter" {
          w456 = u8 1  # length
          n151 = Build Array(w455, w454, w453, w456, u8 44 ("code")) -> (w449:u8[])
          n152 = for {
            tunnel: w449 -> [w459] mode=indexing
            tunnel: [w458] -> w450 mode=indexing
            n153 = Flatten To String(anything=w459) -> (data string=w458:string)  [unwired: 3 in, 2 out]
          }
          n154 = call "CheckSum19073.vi"("Array"=w449) -> ("data string"=w452:string)  [unwired: 10 in]
          n155 = Concatenate Strings(w450) -> (w451:string)
          n156 = Concatenate Strings(w451, w452) -> (w448:string)
        }
        frame "Remote/Local" {
          w470 = u8 2  # length
          n157 = Build Array(w469, w468, w467, w470, u8 46 ("code"), w466) -> (w462:u8[])
          n158 = for {
            tunnel: w462 -> [w473] mode=indexing
            tunnel: [w472] -> w463 mode=indexing
            n159 = Flatten To String(anything=w473) -> (data string=w472:string)  [unwired: 3 in, 2 out]
          }
          n160 = call "CheckSum19073.vi"("Array"=w462) -> ("data string"=w465:string)  [unwired: 10 in]
          n161 = Concatenate Strings(w463) -> (w464:string)
          n162 = Concatenate Strings(w464, w465) -> (w461:string)
        }
        frame "Result" {
          w483 = u8 177  # code
          w484 = u8 3  # length
          n163 = Unbundle By Name(w489) -> ("Step"=w482:u8, "Byte"=w488:bool[])
          n164 = Boolean Array To Number(Boolean array=w488) -> (number=w481:u32)
          n165 = To Unsigned Byte Integer(number=w481) -> (unsigned 8bit integer=w480:u8)
          n166 = Build Array(w487, w486, w485, w484, w483, w482, w480) -> (w476:u8[])
          n167 = for {
            tunnel: w476 -> [w491] mode=indexing
            tunnel: [w490] -> w477 mode=indexing
            n168 = Flatten To String(anything=w491) -> (data string=w490:string)  [unwired: 3 in, 2 out]
          }
          n169 = call "CheckSum19073.vi"("Array"=w476) -> ("data string"=w479:string)  [unwired: 10 in]
          n170 = Concatenate Strings(w477) -> (w478:string)
          n171 = Concatenate Strings(w478, w479) -> (w475:string)
        }
      }
    }
  }
  n172 = flat-sequence {
    tunnel: [w493] -> w34
    tunnel: [w492] -> w33
    tunnel: w29 -> [w492]
    tunnel: w34 -> [w497]
    tunnel: w33 -> [w496]
    tunnel: [w495] -> w32
    tunnel: [w494] -> w31
    tunnel: w32 -> [w503]
    tunnel: w31 -> [w502]
    tunnel: w30 -> [w501]
    tunnel: [w500] -> w4
    tunnel: [w499] -> w2
    tunnel: w4 -> [w506]
    tunnel: [w506] -> w3
    tunnel: w2 -> [w505]
    tunnel: [w505] -> w1
    tunnel: w3 -> [w512]
    tunnel: w1 -> [w511]
    tunnel: [w510] -> _
    tunnel: [w509] -> w5
    tunnel: [w507] -> w8
    tunnel: [w508] -> w10
    frame #0 {
      n173 = global read "meter global.vi" "19073 485 port"() -> (w493:refnum<visa-resource-name>)
    }
    frame #1 {
      n174 = VISA Flush I/O Buffer(VISA resource name=w497, error in (no error)=w496) -> (VISA resource name out=w494:refnum<visa-resource-name>, error out=w495:errorcluster)  [unwired: 1 in]
    }
    frame #2 {
      n175 = VISA Write(VISA resource name=w502, write buffer=w501, error in (no error)=w503) -> (VISA resource name out=w500:refnum<visa-resource-name>, error out=w499:errorcluster)  [unwired: 1 out]
      n176 = Wait Until Next ms Multiple(millisecond multiple=u32 20) -> ()  [unwired: 1 out]
    }
    frame #3 {
      n177 = Wait (ms)(milliseconds to wait=u32 111) -> ()  [unwired: 1 out]
    }
    frame #4 {
      n178 = Tick Count (ms)() -> (millisecond timer value=w514:u32)
      n179 = while {
        shift-right: [w521] -> w507
        shift-left: "" -> [w516]
        tunnel: w514 -> [w517]
        tunnel: [w526] -> w508
        tunnel: w512 -> [w525]
        tunnel: w511 -> [w524]
        tunnel: [w523] -> w510
        tunnel: [w522] -> w509
        tunnel: [w519] -> _
        stop <- w520 stop-if-true
        w539 = 5.0 ("y")
        n180 = Tick Count (ms)() -> (millisecond timer value=w518:u32)
        n181 = property class="Instr"(reference=w525, error in=w524) -> (reference out=w534:refnum<visa-resource-name>, error out=w533:errorcluster, "Serial Settings:Number of Bytes at Serial Port"=w532:u32)
        n182 = Subtract(x=w518, y=w517) -> (x-y=w529:u32)
        n183 = Wait (ms)(milliseconds to wait=u32 22) -> ()  [unwired: 1 out]
        n184 = VISA Read(VISA resource name=w534, byte count=w532, error in (no error)=w533) -> (VISA resource name out=w523:refnum<visa-resource-name>, read buffer=w530:string, error out=w522:errorcluster)  [unwired: 1 out]
        n185 = Concatenate Strings(w516, w530) -> (w521:string)
        n186 = String Length(string=w516) -> (length=w537:i32)
        n187 = String Subset(string=w516, offset (0)=3, length (rest)=1 ("length (rest)")) -> (substring=w541:string)
        n188 = Unflatten From String(type=u8 0, binary string=w541) -> (value=w515:u8, error out=w519:errorcluster)  [unwired: 3 in, 1 out]
        n189 = Add(x=w515, y=w539) -> (x+y=w536:dbl)
        n190 = Equal?(x=w537, y=w536) -> (x = y?=w535:bool)
        n191 = Not Equal?(x=w536, y=w539) -> (x != y?=w538:bool)
        n192 = And(x=w535, y=w538) -> (x .and. y?=w527:bool)
        n193 = Greater?(x=w529, y="Int_Port Timeout") -> (0:w526:bool)
        n194 = Or(x=w527, y=w526) -> (x .or. y?=w520:bool)
      }
    }
  }
  n195 = flat-sequence {
    tunnel: w5 -> [_]
    tunnel: [w544] -> w23
    frame #0 {
      n196 = Tick Count (ms)() -> (millisecond timer value=w544:u32)
    }
  }
  n197 = String Length(string=w8) -> (length=w16:i32)
  n198 = Tick Count (ms)() -> (millisecond timer value=w24:u32)
  n199 = expression code="x-1"(w16) -> (w13:i32)
  n200 = Subtract(x=w23, y=w24) -> (x-y=→"Time_SendNReceive":u32)
  n201 = String Subset(string=w8, offset (0)=w13, length (rest)=1 ("length (rest)")) -> (substring=w11:string)
  n202 = for {
    N: w13 -> [_]
    tunnel: w8 -> [w551]
    tunnel: [w546] -> w15 mode=indexing
    tunnel: [w545] -> _
    i -> [w550]
    n203 = String Subset(string=w551, offset (0)=w550, length (rest)=1 ("length (rest)")) -> (substring=w548:string)
    n204 = Unflatten From String(type=u8 0, binary string=w548) -> (value=w546:u8, error out=w545:errorcluster)  [unwired: 3 in, 1 out]
  }
  n205 = call "CheckSum19073.vi"("Array"=w15) -> ("data string"=w14:string)  [unwired: 10 in]
  n206 = Equal?(x=w14, y=w11) -> (x = y?=w7:bool)
  n207 = case shown="False" w10 {
    tunnel: [w558 Enum_ErrorType."ComError"] -> w9
    tunnel: w8 -> [w553 _]
    frame False {
      n208 = String Subset(string=w553, offset (0)=5, length (rest)=1 ("length (rest)")) -> (substring=w556:string)
      n209 = Unflatten From String(type=u8 0, binary string=w556) -> (value=w552:u8)  [unwired: 3 in, 2 out]
      n210 = case shown="0, Default" w552 {
        tunnel: [Enum_ErrorType."Command Error" Enum_ErrorType."Parameter Error" Enum_ErrorType."OK"] -> w558
        frame 1 {
        }
        frame 2 {
        }
        frame 0, Default {
        }
      }
    }
    frame True {
    }
  }
  "Enum_ErrorType" <- w9
  n211 = Not(x=w7) -> (.not. x?=→"ChecksumError":bool)
  "Boolean_ComErr" <- w10
  "Str_ ReplyStr" <- w8
  "ErrOut" <- w5
